vi "g.vi"(11 "Experiment Parameters From 1st ITX":T1) -> ()   [LabVIEW 2016]
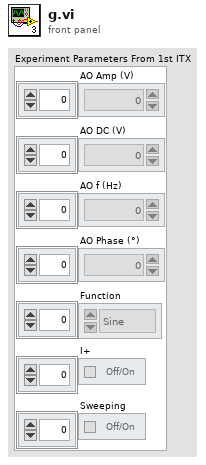
[diagram p1: front panel]
types:
  T1 = cluster{"AO Amp (V)":dbl[], "AO DC (V)":dbl[], "AO f (Hz)":dbl[], "AO Phase (°)":dbl[], "Function":enum16{"Sine", "Triangle", "Square", "Sawtooth"}[], "I+":bool[], "Sweeping":bool[]}
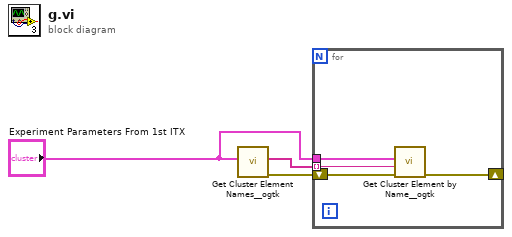
[diagram p0: block diagram]
diagram:
  n1 = call <userlib>:"Get Cluster Element Names__ogtk.vi"("Cluster"="Experiment Parameters From 1st ITX") -> ("error out"=w3:errorcluster, "Element Names"=w1:string[])  [unwired: 9 in]
  n2 = for {
    tunnel: w1 -> [w7] mode=indexing
    tunnel: "Experiment Parameters From 1st ITX" -> [w6]
    shift-right: [w4] -> _
    shift-left: w3 -> [w5]
    n3 = call <userlib>:"Get Cluster Element by Name__ogtk.vi"("error in (no error)"=w5, "Element Name"=w7, "Cluster"=w6) -> ("error out"=w4:errorcluster)  [unwired: 6 in, 2 out]
  }
